vi "PUT Save Directory.vi"(0 "Save Directory":path) -> ()   [LabVIEW 2013]
uses:
  Action.ctl
  Persistent Data FGV Selector.ctl
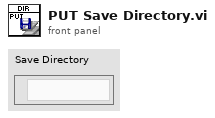
[diagram p1: front panel]
types:
  T1 = typedef "Persistent Data FGV Selector.ctl" = enum16{"Save Directory", "File Name"}
  T2 = typedef "Action.ctl" = enum16{"GET", "PUT", "DELETE"}
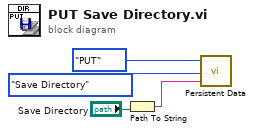
[diagram p0: block diagram]
diagram:
  n1 = Path To String(path="Save Directory") -> (string=w1:string)
  n2 = call "Persistent Data.vi"("Input"=w1, "Persistent Data FGV Selector"=Persistent_Data_FGV_Selector."Save Directory", "Action"=Action."PUT") -> ()  [unwired: 1 out]
